vi "Agilent E3633A Apply Current.vi"(6 "error in (no error)":errorcluster {"code" format="%.0x"}, 8 "Current [A]":dbl format="%.3f", 9 "resource name":refnum<k15>="GPIB0::5::INSTR") -> (0 "error out":errorcluster {"code" format="%.0x"}, 3 "instrument handle out":refnum<k15>)   [LabVIEW 2016]
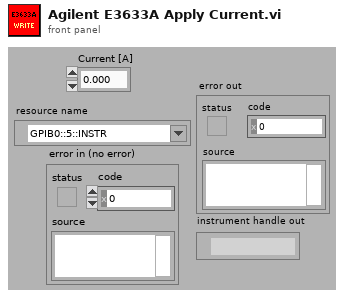
[diagram p1: front panel]
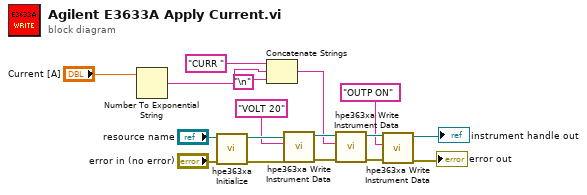
[diagram p0: block diagram]
diagram:
  n1 = Number To Exponential String(number="Current [A]") -> (E-format string=w7:string)  [unwired: 3 in]
  n2 = call "hpe363xa Initialize.vi"("error in (no error)"="error in (no error)", "resource name"="resource name") -> ("error out"=w11:errorcluster, "instrument handle out"=w12:refnum<k15>)  [unwired: 8 in]
  n3 = Concatenate Strings("CURR " ("write CURR Buff"), w7, "\n") -> (w15:string)
  n4 = call "hpe363xa Write Instrument Data.vi"("error in (no error)"=w11, "Write Buffer"="VOLT 20" ("write VOLT Buff"), "instrument handle"=w12) -> ("error out"=w16:errorcluster, "instrument handle out"=w17:refnum<k15>)  [unwired: 7 in]
  n5 = call "hpe363xa Write Instrument Data.vi"("error in (no error)"=w16, "Write Buffer"=w15, "instrument handle"=w17) -> ("error out"=w4:errorcluster, "instrument handle out"=w5:refnum<k15>)  [unwired: 7 in]
  n6 = call "hpe363xa Write Instrument Data.vi"("error in (no error)"=w4, "Write Buffer"="OUTP ON" ("Turn ON Output"), "instrument handle"=w5) -> ("error out"=→"error out":errorcluster, "instrument handle out"=→"instrument handle out":refnum<k15>)  [unwired: 7 in]
